vi "Create DSFChannel.vi"(8 "error in (no error)":errorcluster, 9 "DSFChannel info":T1, 10 "id":string, 11 "DSFChannel in":refnum<class "DSFChannel.lvclass">) -> (0 "error out":errorcluster, 3 "DSFChannel out":refnum<class "DSFChannel.lvclass">)   [LabVIEW 2017, in "DSFChannel.lvclass"]
uses:
  DSFChannel.lvclass
  DSFChannel.lvclass/DSFChannel.ctl
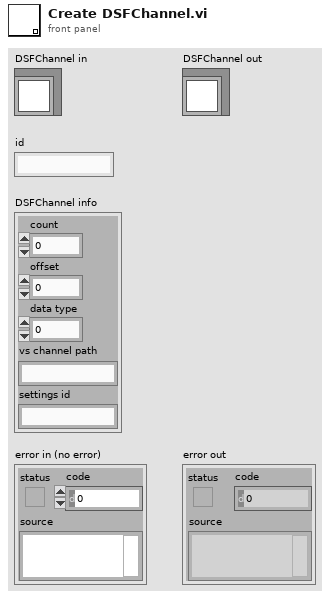
[diagram p1: front panel]
types:
  T1 = cluster{"count":i32, "offset":i32, "data type":i32, "vs channel path":string, "settings id":string}
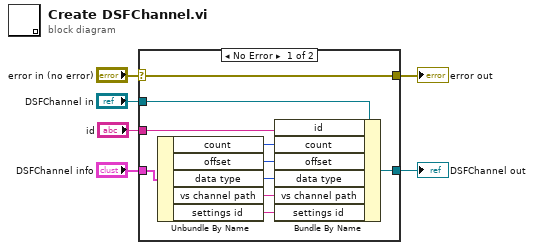
[diagram p0: block diagram]
diagram:
  n1 = case shown="No Error" "error in (no error)" {
    selector: "error in (no error)" -> [w8 w18]
    tunnel: [w8 w18] -> w5
    tunnel: [w9 w17] -> w3
    tunnel: "DSFChannel in" -> [w15 w17]
    tunnel: "DSFChannel info" -> [w16 _]
    tunnel: "id" -> [w7 _]
    frame No Error {
      n2 = Unbundle By Name(w16) -> ("count"=w14:i32, "offset"=w13:i32, "data type"=w12:i32, "vs channel path"=w11:string, "settings id"=w10:string)
      n3 = Bundle By Name(cluster=w15, "id"=w7, "count"=w14, "offset"=w13, "data type"=w12, "vs channel path"=w11, "settings id"=w10) -> (w9:refnum<class "DSFChannel.lvclass">)
    }
    frame Error {
    }
  }
  "error out" <- w5
  "DSFChannel out" <- w3
